vi "Bundle Into Cluster.vi"(8 "error in":errorcluster, 10 "Cluster Elements in":variant[](array[variant])) -> (0 "error out":errorcluster, 2 "Cluster Out":variant)   [LabVIEW 2024, in "Generic Config Handling.lvlib"]
doc: "This vi takes an array of variants and converts them into a variant which represents a cluster."
uses:
  Generic Config Handling.lvlib
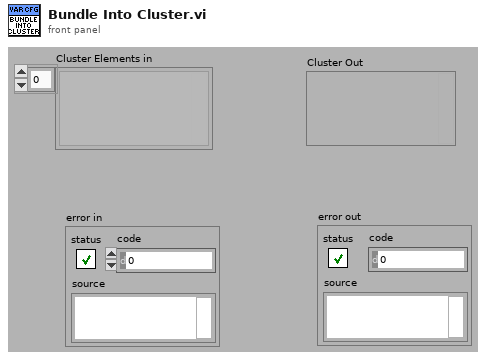
[diagram p1: front panel]
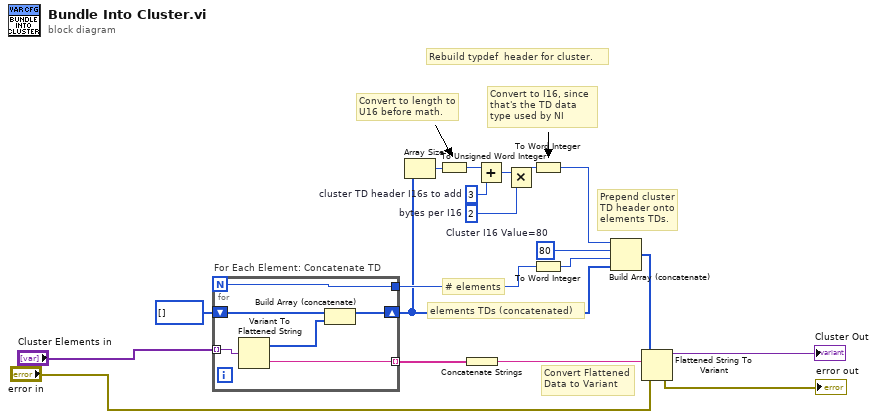
[diagram p0: block diagram]
diagram:
  w1 = i16 80  # Cluster I16 Value=80
  w13 = u16 2  # bytes per I16
  w11 = u16 3  # cluster TD header I16s to add
  # "Rebuild typdef  header for cluster."
  # "Convert Flattened Data to Variant"
  # "elements TDs (concatenated)"
  # "Convert to length to U16 before math."
  # "Convert to I16, since that's the TD data type used by NI"
  # "Prepend cluster TD header onto elements TDs."
  # "# elements"
  n1 = for "For Each Element: Concatenate TD" {
    N -> [w20]
    tunnel: "Cluster Elements in" -> [w25] mode=indexing
    tunnel: [w24] -> w2 mode=indexing
    shift-right: [w22] -> w8
    shift-left: i16[] [] -> [w21]
    tunnel: [w20] -> w10
    n2 = Variant To Flattened String(Variant=w25) -> (data string=w24:string, 1:w23:i16[])
    n3 = Build Array (concatenate)(w21, w23) -> (w22:i16[])
  }
  n4 = Array Size(array=w8) -> (size(s)=w6:i32)
  n5 = To Unsigned Word Integer(number=w6) -> (unsigned 16bit integer=w14:u16)
  n6 = Concatenate Strings(w2) -> (w4:string)
  n7 = Add(x=w14, y=w11) -> (x+y=w12:u16)
  n8 = Multiply(x=w12, y=w13) -> (x*y=w15:u16)
  n9 = To Word Integer(number=w15) -> (16bit integer=w7:i16)
  n10 = To Word Integer(number=w10) -> (16bit integer=w9:i16)
  n11 = Build Array (concatenate)(w7, w1, w9, w8) -> (w5:i16[])
  n12 = Flattened String To Variant(4:"error in", 6:w4, 7:w5) -> (0:→"error out":errorcluster, 3:→"Cluster Out":variant)
